vi "Main.vi"   [LabVIEW 2018]
uses:
  OfficeTron3000/OfficeTron3000.lvclass
  IPrinter/IPrinter.lvclass
  OT3IPrinter/OT3IPrinter.lvclass
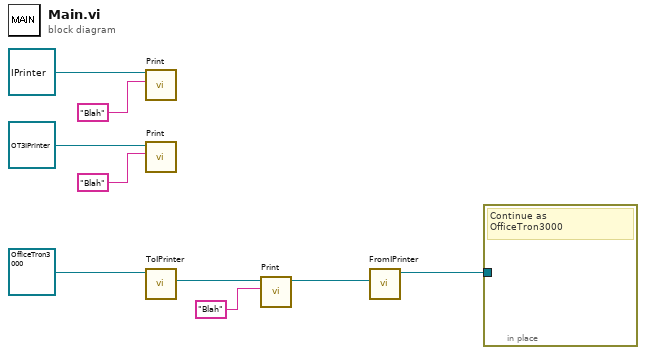
[diagram p0: block diagram]
diagram:
  n1 = call-dynamic "Print.vi"("String"="Blah", "IPrinter In"=refnum<class "IPrinter.lvclass"> refnum ("IPrinter.lvclass")) -> ()  [unwired: 9 in, 1 out]
  n2 = call-dynamic "Print.vi"("String"="Blah", "OT3IPrinter In"=refnum<class "OT3IPrinter.lvclass"> refnum ("OfficeTron3000.lvlib:OT3IPrinter.lvclass")) -> ()  [unwired: 9 in, 1 out]
  n3 = call "ToIPrinter.vi"("OfficeTron3000"=refnum<class "OfficeTron3000.lvclass"> refnum ("OfficeTron3000.lvlib:OfficeTron3000.lvclass")) -> ("OT3IPrinter"=w8:refnum<class "OT3IPrinter.lvclass">)  [unwired: 10 in]
  n4 = call-dynamic "Print.vi"("String"="Blah", "OT3IPrinter In"=w8) -> ("OT3IPrinter Out"=w7:refnum<class "OT3IPrinter.lvclass">)  [unwired: 9 in]
  n5 = call "FromIPrinter.vi"("OT3IPrinter"=w7) -> ("OfficeTron3000"=w6:refnum<class "OfficeTron3000.lvclass">)  [unwired: 10 in]
  n6 = in-place {
    in-place-border: w6 -> [_]
    # "Continue as \nOfficeTron3000"
  }
